vi "GetEnchantment.vi"(8 "Error In":errorcluster, 11 "reference in":refnum<class "Hammer.lvclass">) -> (0 "Error Out":errorcluster, 2 "Return(LabVIEW Class)":refnum<class "IEnchantment.lvclass">, 3 "reference out":refnum<class "Hammer.lvclass">)   [LabVIEW 2020, in "Hammer.lvclass"]
uses:
  Hammer.lvclass
  Hammer.lvclass/Hammer.ctl
  IEnchantment_interface/IEnchantment.lvclass
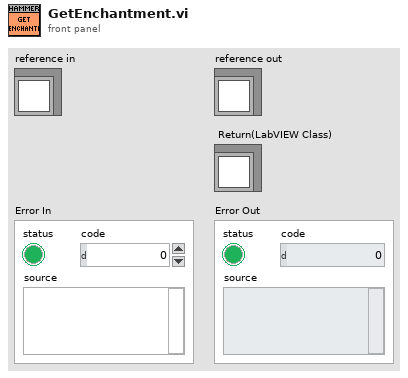
[diagram p1: front panel]
types:
  T1 = typedef "Hammer.lvclass/ObjectAttributes.ctl" = cluster{"_enchantment":refnum<class "IEnchantment.lvclass">}
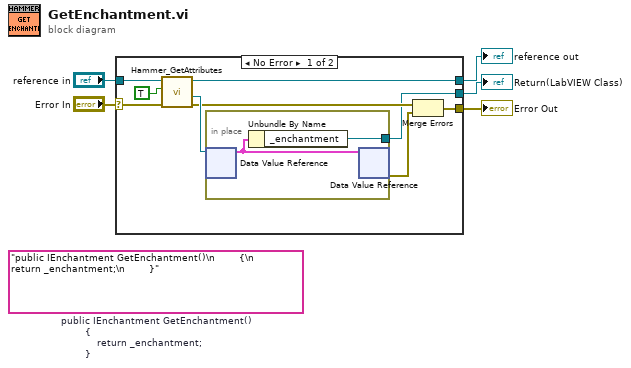
[diagram p0: block diagram]
diagram:
  (unwired) "public IEnchantment GetEnchantment()\n        {\n            return _enchantment;\n        }"  # public IEnchantment GetEnchantment()         {             return _enchantment;         }
  n1 = case shown="No Error" "Error In" {
    selector: "Error In" -> [w13 w18]
    tunnel: [w10 w18] -> w4
    tunnel: [w11 w17] -> w2
    tunnel: "reference in" -> [w14 w17]
    tunnel: [w6 _] -> w1
    frame No Error {
      n2 = call "Hammer_GetAttributes.vi"("error in (no error)"=w13, "OnlyGetDvrReference(False)"=TRUE, "reference in"=w14) -> ("error out"=w8:errorcluster, "DataRef"=w9:refnum<data-value>, "reference out"=w11:refnum<class "Hammer.lvclass">)  [unwired: 5 in, 1 out]
      n3 = in-place {
        in-place-border: [w16] -> w6
        n4 = in-place-dvr #1(w9) -> (w15:T1)  [unwired: 1 out]
        n5 = Unbundle By Name(w15) -> ("_enchantment"=w16:refnum<class "IEnchantment.lvclass">)
        n6 = in-place-dvr #1(w15) -> (w12:errorcluster)  [unwired: 1 out]
      }
      n7 = Merge Errors(w8, w12) -> (w10:errorcluster)
    }
    frame Error {
    }
  }
  "Error Out" <- w4
  "reference out" <- w2
  "Return(LabVIEW Class)" <- w1
